vi "SPC_SetUP.vi"(8 "error in (no error)":errorcluster {"code" format="%.0x"}, 10 "PC":T1={"Number of Bins"=100, "Bin Time (s)"=0.1, "Pause Time (s)"=1e-06}, 11 "VISA Refnum in":refnum<visa-resource-name>) -> (0 "error out":errorcluster {"code" format="%.0x"}, 3 "VISA Refnum out":refnum<visa-resource-name>)   [LabVIEW 2022 SP3]
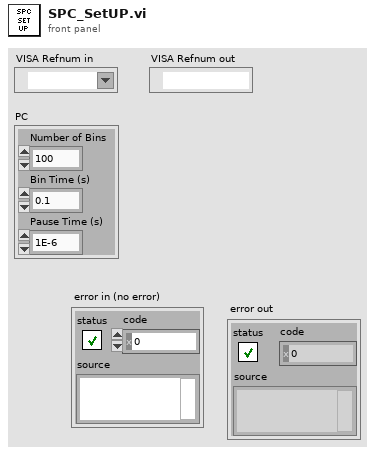
[diagram p1: front panel]
types:
  T1 = cluster{"Number of Bins":i16, "Bin Time (s)":dbl, "Pause Time (s)":dbl}
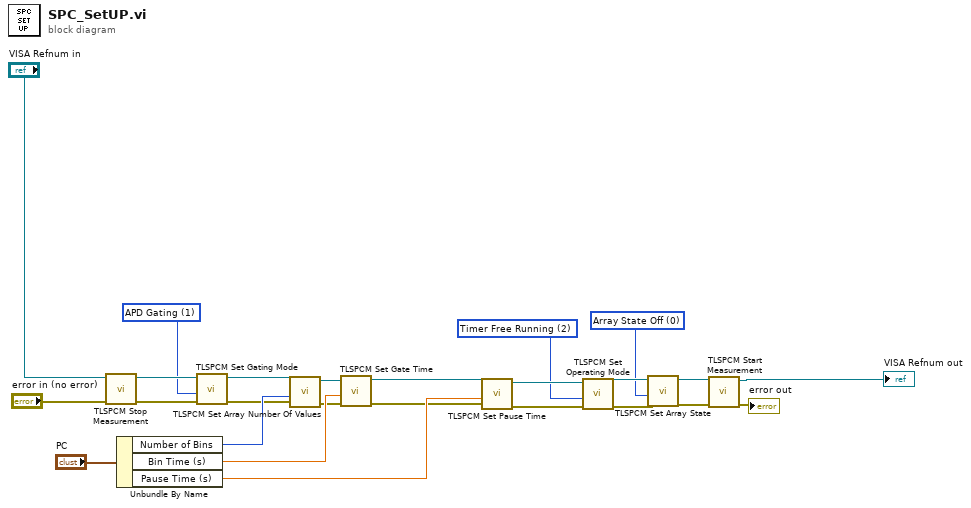
[diagram p0: block diagram]
diagram:
  w4 = u16 0 items=["Array State Off", "Array State On"] ("Set Array State (Array State Off)")
  w5 = i16 2 items=["User Mode"=1, "Timer Free Running"=2, "Triggered by Timer"=3, "Triggered by external Signal"=4, "Gating by External Signal"=5] ("Operating Mode (Triggered by Timer)")
  w13 = i16 1 items=["APD Gating"=1, "Counter Gating"=0] ("Gating Mode (Counter Gating)")
  n1 = call <instrlib>:"TLSPCM Stop Measurement.vi"("error in (no error)"="error in (no error)", "instrument handle"="VISA Refnum in") -> ("error out"=w16:errorcluster, "instrument handle out"=w17:refnum<visa-resource-name>)  [unwired: 8 in]
  n2 = Unbundle By Name("PC") -> ("Number of Bins"=w14:i16, "Bin Time (s)"=w24:dbl, "Pause Time (s)"=w25:dbl)
  n3 = call <instrlib>:"TLSPCM Set Gating Mode.vi"("error in (no error)"=w16, "Gating Mode (Counter Gating)"=w13, "instrument handle"=w17) -> ("error out"=w12:errorcluster, "instrument handle out"=w15:refnum<visa-resource-name>)  [unwired: 7 in]
  n4 = call <instrlib>:"TLSPCM Set Array Number Of Values.vi"("error in (no error)"=w12, "Number of Array Values (100)"=w14, "instrument handle"=w15) -> ("error out"=w19:errorcluster, "instrument handle out"=w18:refnum<visa-resource-name>)  [unwired: 7 in]
  n5 = call <instrlib>:"TLSPCM Set Gate Time.vi"("error in (no error)"=w19, "Gate Time (0.1)"=w24, "instrument handle"=w18) -> ("error out"=w21:errorcluster, "instrument handle out"=w20:refnum<visa-resource-name>)  [unwired: 7 in]
  n6 = call <instrlib>:"TLSPCM Set Pause Time.vi"("error in (no error)"=w21, "Pause Time (0.000001)"=w25, "instrument handle"=w20) -> ("error out"=w10:errorcluster, "instrument handle out"=w11:refnum<visa-resource-name>)  [unwired: 7 in]
  n7 = call <instrlib>:"TLSPCM Set Operating Mode.vi"("error in (no error)"=w10, "Operating Mode (Triggered by Timer)"=w5, "instrument handle"=w11) -> ("error out"=w8:errorcluster, "instrument handle out"=w9:refnum<visa-resource-name>)  [unwired: 7 in]
  n8 = call <instrlib>:"TLSPCM Set Array State.vi"("error in (no error)"=w8, "Set Array State (Array State Off)"=w4, "instrument handle"=w9) -> ("error out"=w6:errorcluster, "instrument handle out"=w7:refnum<visa-resource-name>)  [unwired: 7 in]
  n9 = call <instrlib>:"TLSPCM Start Measurement.vi"("error in (no error)"=w6, "instrument handle"=w7) -> ("error out"=→"error out":errorcluster, "instrument handle out"=→"VISA Refnum out":refnum<visa-resource-name>)  [unwired: 8 in]
